vi "Read Axis Map.vi"(8 "error in (no error)":errorcluster, 11 "Motion Controller in":refnum<class "Parent SIM Motion Controller.lvclass">) -> (0 "error out":errorcluster, 2 "Axis Map":map{string, T1}(c390), 3 "Motion Controller out":refnum<class "Parent SIM Motion Controller.lvclass">)   [LabVIEW 2022 SP3, in "Parent SIM Motion Controller.lvclass"]
uses:
  Parent SIM Motion Controller.lvclass
  Axis Data.ctl
  Axis Parameters.ctl
  Axis Settings.ctl
  Parent SIM Motion Controller.lvclass/Parent SIM Motion Controller.ctl
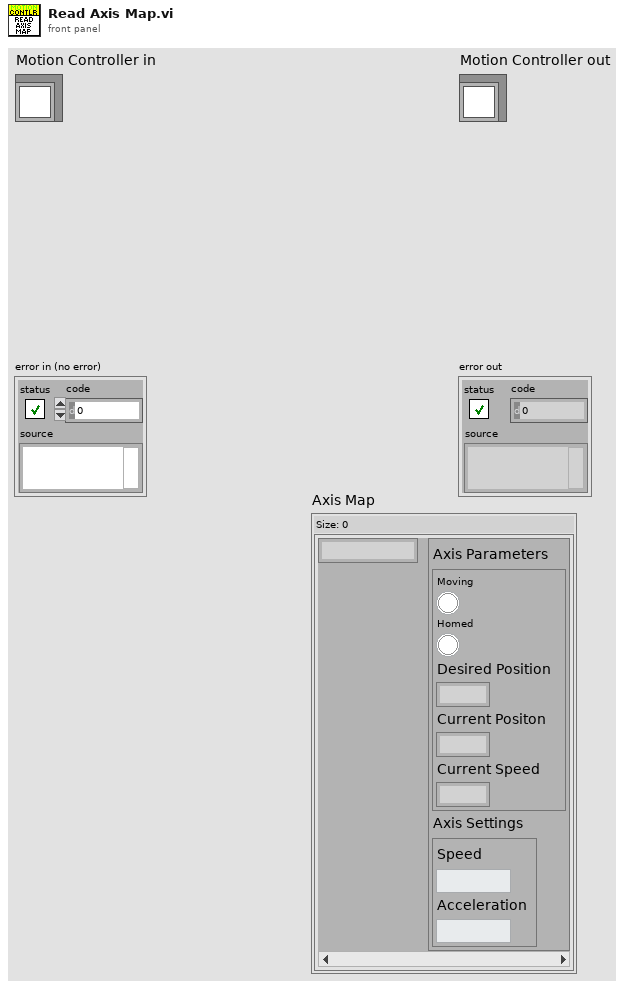
[diagram p1: front panel]
types:
  T1 = typedef "Parent SIM Motion Controller.lvclass/Axis Data.ctl" = cluster{"Axis Parameters":T2, "Axis Settings":T3}
  T2 = typedef "Parent SIM Motion Controller.lvclass/Axis Parameters.ctl" = cluster{"Moving":bool, "Homed":bool, "Desired Position":dbl, "Current Positon":dbl, "Current Speed":dbl}
  T3 = typedef "Parent SIM Motion Controller.lvclass/Axis Settings.ctl" = cluster{"Speed":dbl, "Acceleration":dbl}
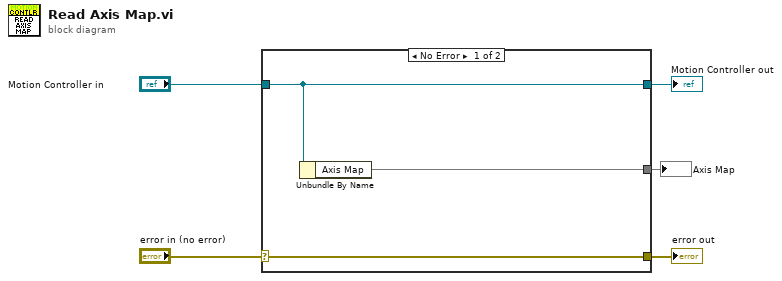
[diagram p0: block diagram]
diagram:
  n1 = case shown="No Error" "error in (no error)" {
    selector: "error in (no error)" -> [w8 w9]
    tunnel: [w8 w9] -> w4
    tunnel: [w7 w10] -> w2
    tunnel: "Motion Controller in" -> [w7 w10]
    tunnel: [w6 _] -> w1
    frame No Error {
      n2 = Unbundle By Name(w7) -> ("Axis Map"=w6:map{string, T1})
    }
    frame Error {
    }
  }
  "error out" <- w4
  "Motion Controller out" <- w2
  "Axis Map" <- w1
